vi "CreateMainMenu.vi"(11 "菜单输入":refnum<k9>) -> ()   [LabVIEW 2015]
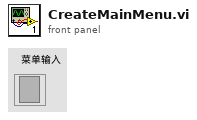
[diagram p1: front panel]
types:
  T1 = cluster{"MenuNames":string[], "MenuTags":string[]}
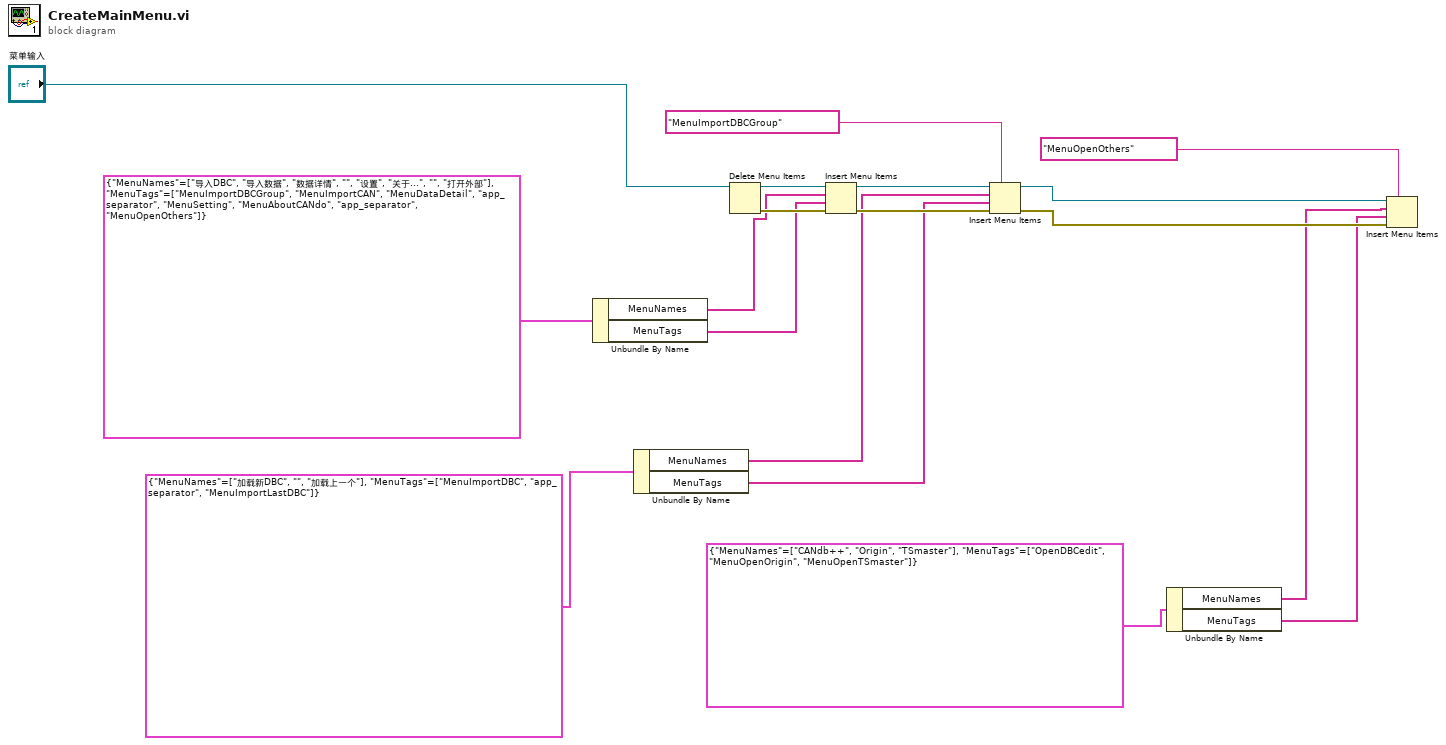
[diagram p0: block diagram]
diagram:
  n1 = Unbundle By Name(T1 {"MenuNames"=["导入DBC", "导入数据", "数据详情", "", "设置", "关于...", "", "打开外部"], "MenuTags"=["MenuImportDBCGroup", "MenuImportCAN", "MenuDataDetail", "app_separator", "MenuSetting", "MenuAboutCANdo", "app_separator", "MenuOpenOthers"]}) -> ("MenuNames"=w8:string[], "MenuTags"=w7:string[])
  n2 = Unbundle By Name(T1 {"MenuNames"=["加载新DBC", "", "加载上一个"], "MenuTags"=["MenuImportDBC", "app_separator", "MenuImportLastDBC"]}) -> ("MenuNames"=w4:string[], "MenuTags"=w5:string[])
  n3 = Delete Menu Items(9:"菜单输入") -> (0:w18:errorcluster, 3:w14:refnum<k9>)  [unwired: 3 in]
  n4 = Insert Menu Items(6:w18, 7:w7, 8:w8, 9:w14) -> (0:w16:errorcluster, 3:w10:refnum<k9>)  [unwired: 2 in, 1 out]
  n5 = Insert Menu Items(5:"MenuImportDBCGroup" ("L10n_menu tag"), 6:w16, 7:w5, 8:w4, 9:w10) -> (0:w17:errorcluster, 3:w11:refnum<k9>)  [unwired: 1 in, 1 out]
  n6 = Unbundle By Name(T1 {"MenuNames"=["CANdb++", "Origin", "TSmaster"], "MenuTags"=["OpenDBCedit", "MenuOpenOrigin", "MenuOpenTSmaster"]}) -> ("MenuNames"=w2:string[], "MenuTags"=w1:string[])
  n7 = Insert Menu Items(5:"MenuOpenOthers" ("L10n_menu tag"), 6:w17, 7:w1, 8:w2, 9:w11) -> ()  [unwired: 1 in, 3 out]
